vi "Init SGM31323.vi"(8 "error in (no error)":errorcluster, 11 "I2C RGB SGM31323 in":refnum<class "Grove I2C RGB SGM31323.lvclass">) -> (0 "error out":errorcluster, 3 "I2C RGB SGM31323 out":refnum<class "Grove I2C RGB SGM31323.lvclass">)   [LabVIEW 2020, in "CTI-Peripheral.lvlib" / "Grove I2C RGB SGM31323.lvclass"]
uses:
  Grove I2C RGB SGM31323.lvclass
  Grove I2C RGB SGM31323.lvclass/Grove I2C RGB SGM31323.ctl
  CTI/I2C Connection/I2C Connection.lvclass/I2C Connection.ctl
  CTI/Session/I2C Write Data.vi
  CTI/I2C Connection/I2C Connection.lvclass
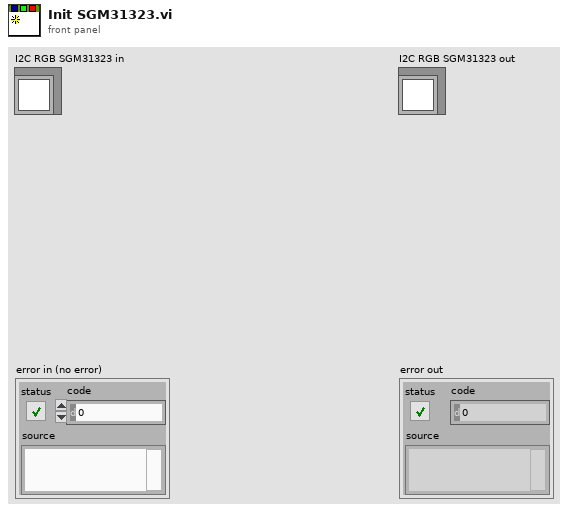
[diagram p1: front panel]
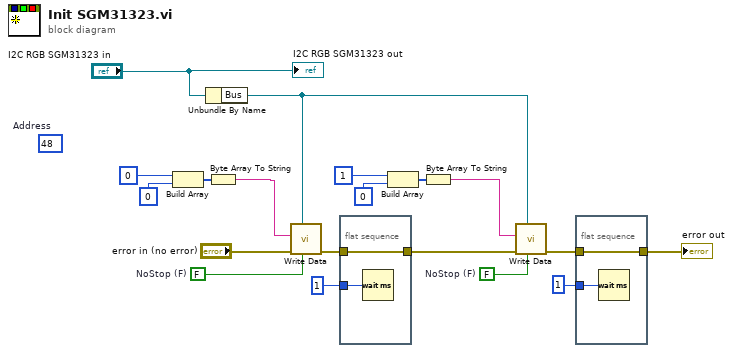
[diagram p0: block diagram]
diagram:
  w8 = FALSE  # NoStop (F)
  w11 = FALSE  # NoStop (F)
  (unwired) u8 48  # Address
  n1 = Build Array(u8 0 ("Value"), u8 0 ("Value")) -> (w16:u8[])
  n2 = Unbundle By Name("I2C RGB SGM31323 in") -> ("Bus"=w18:refnum<class "I2C Connection.lvclass">)
  n3 = Byte Array To String(unsigned byte array=w16) -> (string=w10:string)
  n4 = call "Write Data.vi"("NoStop (F)"=w11, "I2C Connection"=w18, "error in (no error)"="error in (no error)", "Data"=w10) -> ("error out"=w6:errorcluster)  [unwired: 7 in]
  n5 = flat-sequence {
    tunnel: w6 -> [w21]
    tunnel: [w21] -> w5
    tunnel: u32 1 ("milliseconds to wait") -> [w20]
    frame #0 {
      n6 = Wait (ms)(milliseconds to wait=w20) -> ()  [unwired: 1 out]
    }
  }
  n7 = Build Array(u8 1 ("Value"), u8 0 ("Value")) -> (w13:u8[])
  n8 = Byte Array To String(unsigned byte array=w13) -> (string=w7:string)
  n9 = call "Write Data.vi"("NoStop (F)"=w8, "I2C Connection"=w18, "error in (no error)"=w5, "Data"=w7) -> ("error out"=w3:errorcluster)  [unwired: 7 in]
  n10 = flat-sequence {
    tunnel: w3 -> [w23]
    tunnel: [w23] -> w2
    tunnel: u32 1 ("milliseconds to wait") -> [w22]
    frame #0 {
      n11 = Wait (ms)(milliseconds to wait=w22) -> ()  [unwired: 1 out]
    }
  }
  "error out" <- w2
  "I2C RGB SGM31323 out" <- "I2C RGB SGM31323 in"
